vi "Choose JSON Schema Dialect.vi"(8 "error in (no error)":errorcluster, 9 "Custom Dialect":string, 10 "Dialect":T1, 11 "JSON Schema in":string="{}") -> (0 "error out":errorcluster, 3 "JSON Schema out":string="{}")   [LabVIEW 2019, in "JSON-Schema.lvlib"]
doc: "A version of JSON Schema is called a dialect. A dialect represents the set of keywords and semantics that can be used to evaluate a schema. Each JSON Schema release is a new dialect of JSON Schema. JSON Schema provides a way for you to declare which dialect a schema conforms to and provides ways to describe your own custom dialects.\n\nDefault <b>Dialect</b> is <b>2012-12</b>\n\nhttps://json-schema.org/understanding-json-schema/reference/schema#declaring-a-dialect"
uses:
  JSON-Schema.lvlib
  typedefs/JSON Schema Dialect--Enum.ctl
  <vilib>/JDP Science/JSONtext/Get all Object Items.vi
  <vilib>/JDP Science/JSONtext/Set Multiple Object Items.vi
  <vilib>/JDP Science/JSONtext/JSONtext.lvlib
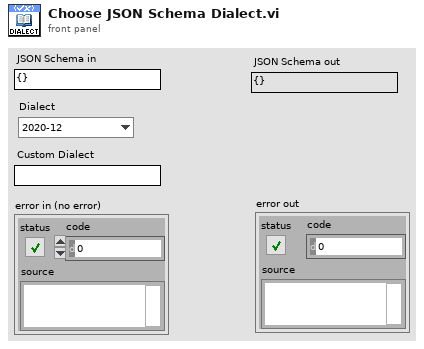
[diagram p1: front panel]
types:
  T1 = typedef "JSON-Schema.lvlib/JSON Schema Dialect--Enum.ctl" = enum16{"2020-12", "2019-09", "draft-07", "draft-06", "draft-05", "custom"}
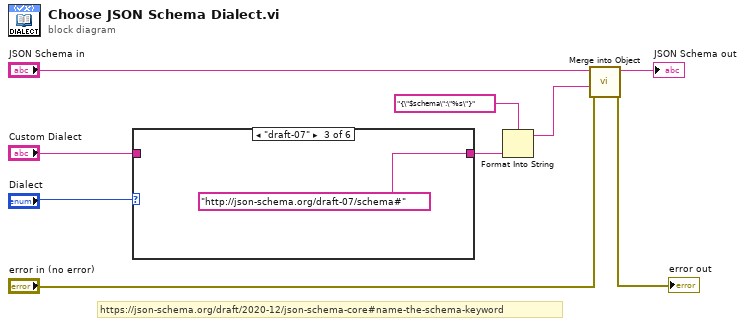
[diagram p0: block diagram]
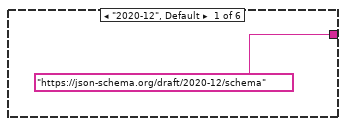
[diagram p2: hidden frame]
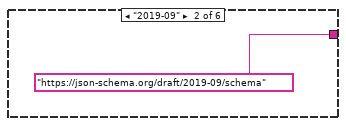
[diagram p3: hidden frame]
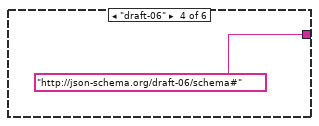
[diagram p4: hidden frame]
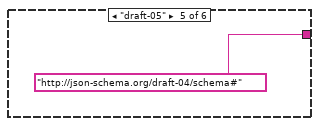
[diagram p5: hidden frame]
diagram:
  # "https://json-schema.org/draft/2020-12/json-schema-core#name-the-schema-keyword"
  n1 = case shown="\"draft-07\"" "Dialect" {
    tunnel: ["https://json-schema.org/draft/2020-12/schema" ("JSON to Insert") "https://json-schema.org/draft/2019-09/schema" ("JSON to Insert") "http://json-schema.org/draft-07/schema#" ("JSON to Insert") "http://json-schema.org/draft-06/schema#" ("JSON to Insert") "http://json-schema.org/draft-04/schema#" ("JSON to Insert") w15] -> w7
    tunnel: "Custom Dialect" -> [_ _ _ _ _ w15]
    frame "2020-12", Default {
    }
    frame "2019-09" {
    }
    frame "draft-07" {
    }
    frame "draft-06" {
    }
    frame "draft-05" {
    }
    frame "custom" {
    }
  }
  n2 = Format Into String(format string="{\"$schema\":\"%s\"}", w7) -> (resulting string=w4:string)  [unwired: 2 in, 1 out]
  n3 = call <vilib>:"Merge into Object.vi"("error in (no error)"="error in (no error)", "JSON Object to Merge"=w4, "JSON"="JSON Schema in") -> ("error out"=→"error out":errorcluster, "<JSON>"=→"JSON Schema out":string)  [unwired: 6 in]
